vi "Cache_Members Global_Load All.vi"(8 "error in (no error)":errorcluster) -> (0 "error out":errorcluster, 1 "All Success?":bool, 3 "All Members":map{string, T1}(c390))   [LabVIEW 2020, in "ClassLoader.lvlib"]
uses:
  ClassLoader.lvlib
  Ctl/Ctl_Member Map.ctl
  <vilib>/Utility/Data Type/Member VI Info.ctl
  Cache_Members Global.vi
  <vilib>/Utility/config.llb/NI_LVConfig.lvlib
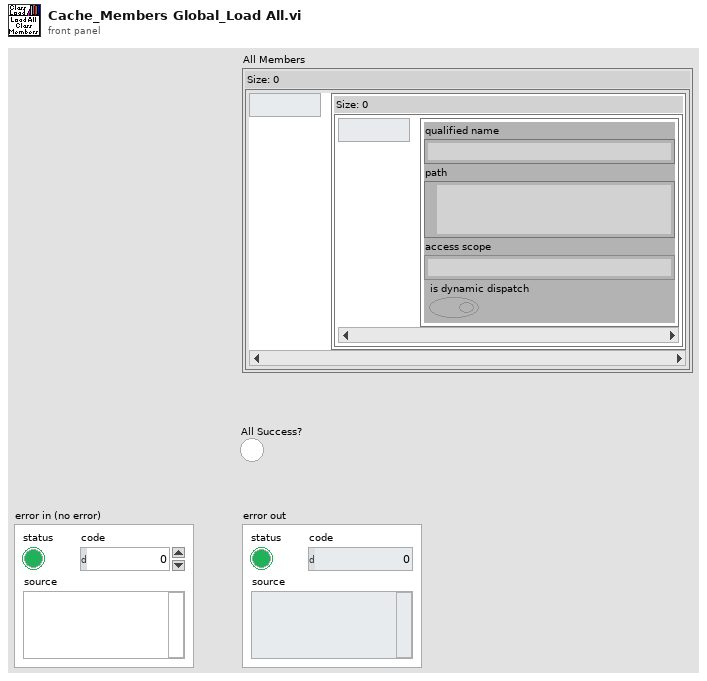
[diagram p1: front panel]
types:
  T1 = typedef "ClassLoader.lvlib/Ctl_Member Map.ctl" = map{string, T2}
  T2 = typedef "Member VI Info.ctl" = cluster{"qualified name":string, "path":path, "access scope":enum32{"invalid scope", "public", "private", "protected", "community"}, "is dynamic dispatch":bool}
  T3 = typedef "NI_LVConfig.lvlib/Config Data RefNum.ctl" = refnum<k1>
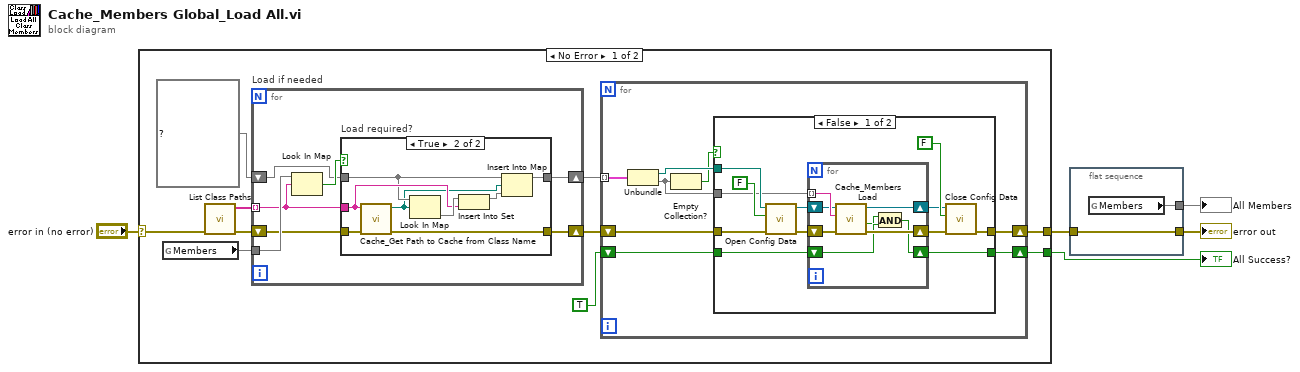
[diagram p0: block diagram]
diagram:
  n1 = case shown="No Error" "error in (no error)" {
    selector: "error in (no error)" -> [w15 w63]
    tunnel: [w9 w63] -> w2
    tunnel: [w6 _] -> w1
    frame No Error {
      n2 = global read "Cache_Members Global.vi" "Members"() -> (w8:map{string, T1})
      n3 = call "List Class Paths.vi"("error in (no error)"=w15) -> ("error out"=w11:errorcluster, "Class Names"=w14:string[])  [unwired: 8 in, 1 out]
      n4 = for "Load if needed" {
        tunnel: w14 -> [w50] mode=indexing
        tunnel: w8 -> [w51]
        shift-right: [w48] -> w10
        shift-left: map{path, set{string}} {} ("map") -> [w49]
        shift-right: [w47] -> w12
        shift-left: w11 -> [w46]
        n5 = Look In Map(map=w51, key=w50) -> (key not found?=w52:bool)  [unwired: 1 in, 1 out]
        n6 = case "Load required?" shown="True" w52 {
          tunnel: w50 -> [_ w61]
          tunnel: w49 -> [w54 w60]
          tunnel: [w54 w59] -> w48
          tunnel: [w53 w55] -> w47
          tunnel: w46 -> [w53 w56]
          frame False {
          }
          frame True {
            n7 = call "Cache_Get Path to Cache from Class Name.vi"("error in (no error)"=w56, "Class Name"=w61) -> ("error out"=w55:errorcluster, "Cache Path"=w58:path)  [unwired: 7 in, 1 out]
            n8 = Look In Map(map=w60, key=w58) -> (value=w62:set{string})  [unwired: 1 in, 1 out]
            n9 = Insert Into Set(10:w61, 11:w62) -> (3:w57:set{string})  [unwired: 1 out]
            n10 = Insert Into Map(map in=w60, key=w58, value=w57) -> (map out=w59:map{path, set{string}})  [unwired: 2 out]
          }
        }
      }
      n11 = for {
        tunnel: w10 -> [w23] mode=indexing
        shift-right: [w20] -> w9
        shift-left: w12 -> [w21]
        shift-right: [w16] -> w6
        shift-left: TRUE -> [w17]
        n12 = Unbundle(w23) -> ("Cache Path"=w22:path, "set"=w19:set{string})
        n13 = Empty Collection?(1:w19) -> (0:w18:bool)
        n14 = case shown="False" w18 {
          tunnel: w22 -> [w34 _]
          tunnel: w21 -> [w33 w45]
          tunnel: [w27 w45] -> w20
          tunnel: w19 -> [w26 _]
          tunnel: w17 -> [w25 w44]
          tunnel: [w24 w44] -> w16
          frame False {
            n15 = call <vilib>:"Open Config Data.vi"("error in (no error)"=w33, "create file if necessary (T)"=FALSE, "configuration file path"=w34) -> ("error out"=w29:errorcluster, "refnum"=w31:T3)  [unwired: 6 in, 1 out]
            n16 = for {
              shift-right: [w41] -> w30
              shift-left: w31 -> [w42]
              tunnel: w26 -> [w43] mode=indexing
              shift-right: [w39] -> w28
              shift-left: w29 -> [w40]
              shift-right: [w36] -> w24
              shift-left: w25 -> [w38]
              n17 = call "Cache_Members Load.vi"("error in (no error)"=w40, "Class Name"=w43, "Refnum in"=w42) -> ("error out"=w39:errorcluster, "Success?"=w37:bool, "Refnum out"=w41:T3)  [unwired: 5 in, 1 out]
              n18 = And(x=w37, y=w38) -> (x .and. y?=w36:bool)
            }
            n19 = call <vilib>:"Close Config Data.vi"("error in (no error)"=w28, "write file if changed (T)"=FALSE, "refnum"=w30) -> ("error out"=w27:errorcluster)  [unwired: 7 in, 1 out]
          }
          frame True {
          }
        }
      }
    }
    frame Error {
    }
  }
  "All Success?" <- w1
  n20 = flat-sequence {
    tunnel: [w65] -> w4
    tunnel: [w64] -> w3
    tunnel: w2 -> [w64]
    frame #0 {
      n21 = global read "Cache_Members Global.vi" "Members"() -> (w65:map{string, T1})
    }
  }
  "error out" <- w3
  "All Members" <- w4
